vi "Auto_Routine_Deposit_Backup_Balance.vi"(8 "error in (no error)":errorcluster, 10 "Game Piece":T1, 11 "Position":T2=enum."Middle") -> (0 "error out":errorcluster)   [LabVIEW 2023]
uses:
  Arm/ArmPositionPreset.ctl
  Arm/ArmGamePiecePreset.ctl
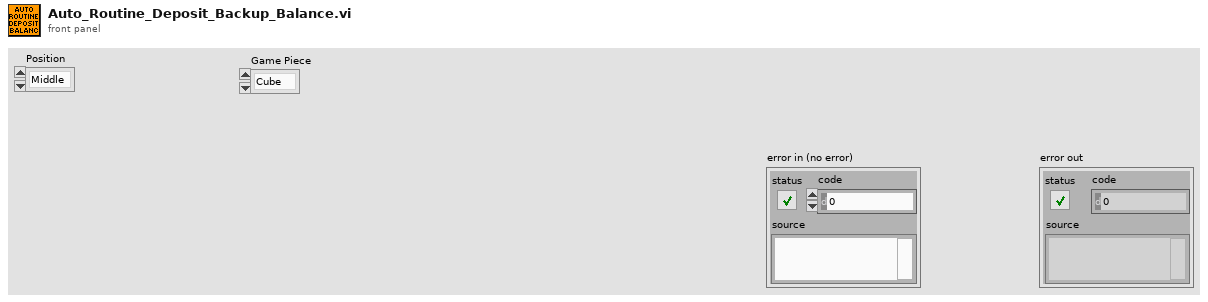
[diagram p1: front panel]
types:
  T1 = typedef "ArmGamePiecePreset.ctl" = enum16{"Cube", "Cone"}
  T2 = typedef "ArmPositionPreset.ctl" = enum16{"Upper", "Lower", "Middle", "Home", "Shelf", "Floor", "HalfFloor", "HalfHome"}
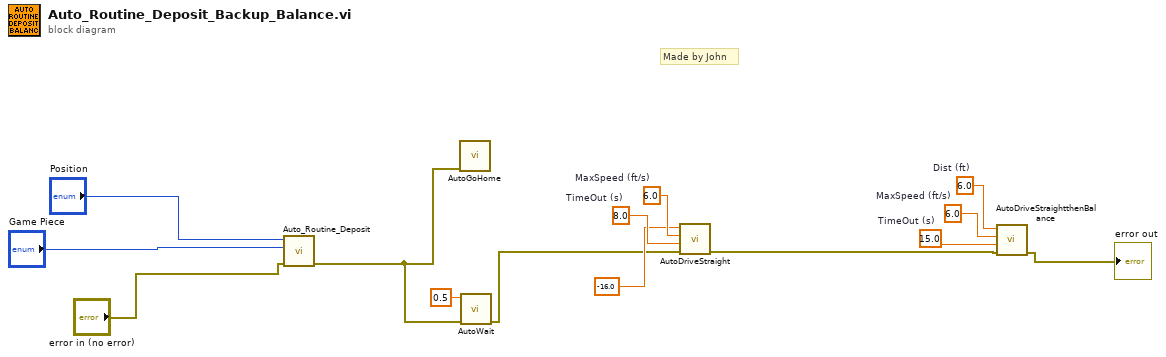
[diagram p0: block diagram]
diagram:
  w9 = 15.0  # TimeOut (s)
  w10 = 6.0  # MaxSpeed (ft/s)
  w11 = 6.0  # Dist (ft)
  w12 = 8.0  # TimeOut (s)
  w13 = 6.0  # MaxSpeed (ft/s)
  # "Made by John"
  n1 = call "Auto_Routine_Deposit.vi"("error in (no error)"="error in (no error)", "Game Piece"="Game Piece", "Position"="Position") -> ("error out"=w2:errorcluster)  [unwired: 8 in]
  n2 = call "AutoGoHome.vi"("error in (no error)"=w2) -> ()  [unwired: 10 in, 1 out]
  n3 = call "AutoWait.vi"("error in (no error)"=w2, "TimeOut (s)"=0.5) -> ("error out"=w1:errorcluster)  [unwired: 9 in]
  n4 = call "AutoDriveStraight.vi"("error in (no error)"=w1, "TimeOut (s)"=w12, "MaxSpeed (ft/s)"=w13, "Dist (ft)"=-16.0) -> ("error out"=w14:errorcluster)  [unwired: 7 in]
  n5 = call "AutoDriveStraightthenBalance.vi"("error in (no error)"=w14, "TimeOut (s)"=w9, "MaxSpeed (ft/s)"=w10, "Dist (ft)"=w11) -> ("error out"=→"error out":errorcluster)  [unwired: 7 in]
